vi "write log.vi"(8 "error in (no error)":errorcluster, 10 "log info":T1, 11 "file":path) -> (0 "error out":errorcluster)   [LabVIEW 2015]
uses:
  log info.ctl
  <vilib>/Utility/file.llb/Write Delimited Spreadsheet (string).vi
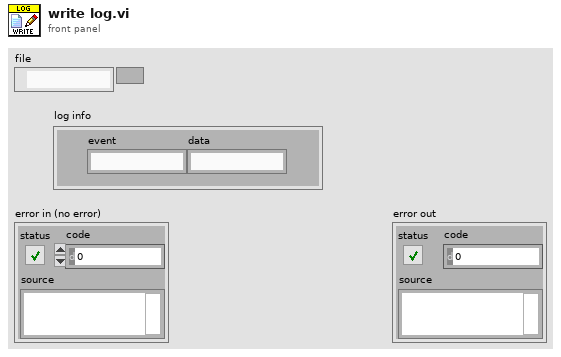
[diagram p1: front panel]
types:
  T1 = typedef "log info.ctl" = cluster{"event":string, "data":string}
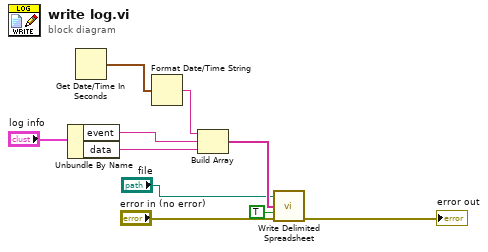
[diagram p0: block diagram]
diagram:
  n1 = Unbundle By Name("log info") -> ("event"=w7:string, "data"=w8:string)
  n2 = Get Date/Time In Seconds() -> (seconds since 1Jan1904=w6:timestamp)
  n3 = Format Date/Time String(seconds (now)=w6) -> (date/time string=w5:string)  [unwired: 2 in]
  n4 = Build Array(w5, w7, w8) -> (w4:string[])
  n5 = call-poly <vilib>:"Write Delimited Spreadsheet.vi"("file path (dialog if empty)"="file", "1D data"=w4, "append to file? (F)"=TRUE, "error in (no error)"="error in (no error)") -> ("error out"=→"error out":errorcluster)  [unwired: 10 in, 1 out]
